vi "test-get-all-encoders.vi"() -> ()   [LabVIEW 2019]
uses:
  <vilib>/Rock Robotics/SystemInterfaces/Encoder/FPGA_EncoderIdx.ctl
panel:
  out "All Encoder Inx":T1[](array[typedef])
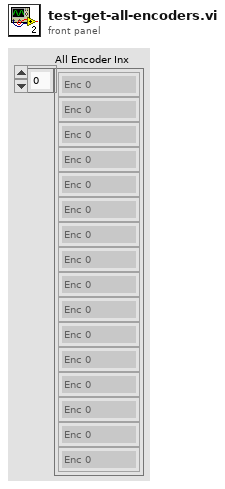
[diagram p1: front panel]
types:
  T1 = typedef "FPGA_EncoderIdx.ctl" = enum8{"Enc 0", "Enc 1", "Enc 2", "Enc 3", "Enc 4", "Enc 5", "Enc 6", "Enc 7", "Invalid"}
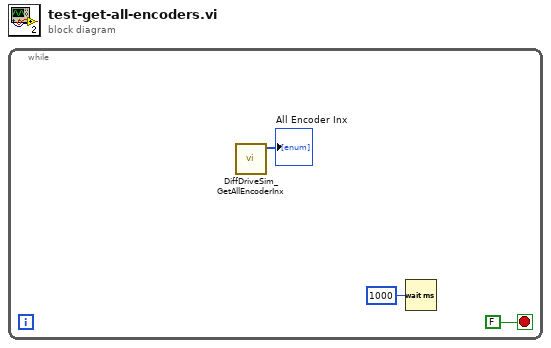
[diagram p0: block diagram]
diagram:
  n1 = while {
    stop <- FALSE stop-if-true
    n2 = call "DiffDriveSim_GetAllEncoderInx.vi"() -> ("All Encoder Inx"=→"All Encoder Inx":T1[])  [unwired: 11 in]
    n3 = Wait (ms)(milliseconds to wait=u32 1000) -> ()  [unwired: 1 out]
  }
